vi "resize FP calc.vi"(9 "Width":u32, 10 "Screen Coordinates":T2, 11 "refs.listbox":refnum<vi>) -> (3 "fp bounds":T1)   [LabVIEW 2021, in "Autocomplete popup.lvlib"]
uses:
  Autocomplete popup.lvlib
  <vilib>/Utility/miscctls.llb/LVPointTypeDef.ctl
  <vilib>/Utility/miscctls.llb/LVRectTypeDef.ctl
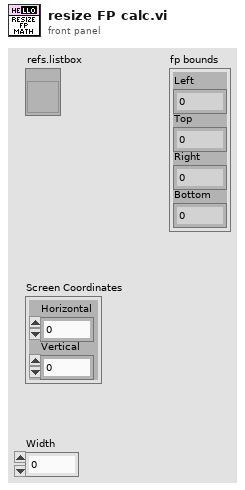
[diagram p1: front panel]
types:
  T1 = typedef "LVRectTypeDef.ctl" = cluster{"Left":i16, "Top":i16, "Right":i16, "Bottom":i16}
  T2 = typedef "LVPointTypeDef.ctl" = cluster{"Horizontal":i16, "Vertical":i16}
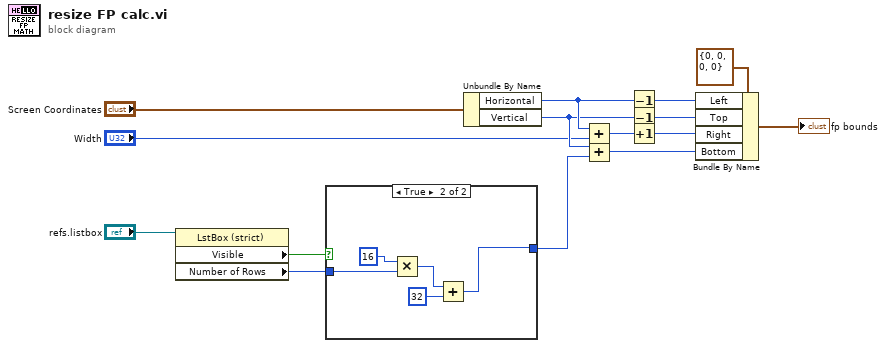
[diagram p0: block diagram]
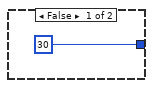
[diagram p2: hidden frame]
diagram:
  n1 = property class="LstBox (strict)"(reference="refs.listbox") -> ("Visible"=w15:bool, "Number of Rows"=w14:u32)  [unwired: 1 in, 2 out]
  n2 = case shown="True" w15 {
    tunnel: w14 -> [_ w20]
    tunnel: [i16 30 ("y") w17] -> w3
    frame False {
    }
    frame True {
      n3 = Multiply(x=i16 16 ("y"), y=w20) -> (x*y=w19:u32)
      n4 = Add(x=w19, y=i16 32) -> (x+y=w17:u32)
    }
  }
  n5 = Unbundle By Name("Screen Coordinates") -> ("Horizontal"=w9:i16, "Vertical"=w8:i16)
  n6 = Add(x=w9, y="Width") -> (x+y=w7:u32)
  n7 = Add(x=w8, y=w3) -> (x+y=w12:u32)
  n8 = Decrement(x=w9) -> (x-1=w11:i16)
  n9 = Decrement(x=w8) -> (x-1=w10:i16)
  n10 = Increment(x=w7) -> (x+1=w6:u32)
  n11 = Bundle By Name(cluster=T1 {"Left"=0, "Top"=0, "Right"=0, "Bottom"=0} ("Bounds"), "Left"=w11, "Top"=w10, "Right"=w6, "Bottom"=w12) -> (→"fp bounds":T1)
